vi "Status.vi"(11 "Sequencer in":refnum<class "Sequencer.lvclass">) -> (2 "Steps":T1[](array[typedef]), 3 "Number Of Steps":i32)   [LabVIEW 2020, in "RTAF.lvlib" / "Sequencer.lvclass"]
uses:
  Sequencer.lvclass
  Single Step Data.ctl
  Sequencer.lvclass/Sequencer.ctl
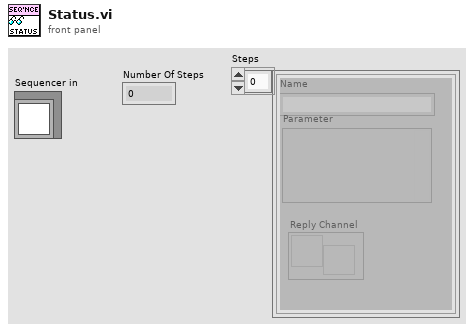
[diagram p1: front panel]
types:
  T1 = typedef "RTAF.lvlib/Sequencer.lvclass/Single Step Data.ctl" = cluster{"Name":string, "Parameter":variant, "Reply Channel":refnum<notifier>}
  T2 = typedef "Sequencer.lvclass/Single Step Data.ctl" = cluster{"Name":string, "Parameter":variant, "Reply Channel":refnum<notifier>}
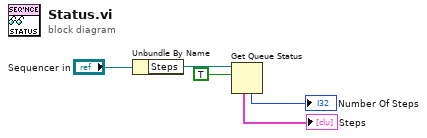
[diagram p0: block diagram]
diagram:
  n1 = Unbundle By Name("Sequencer in") -> ("Steps"=w4:refnum<queue>)
  n2 = Get Queue Status(queue=w4, return elements? (F)=TRUE) -> (# elements in queue=→"Number Of Steps":i32, elements=→"Steps":T2[])  [unwired: 1 in, 6 out]
